vi "Init.vi"(8 "error in (no error)":errorcluster, 11 "PongSwitch in":refnum<class "SnakeSwitch.lvclass">) -> (0 "error out":errorcluster, 3 "PongSwitch out":refnum<class "SnakeSwitch.lvclass">)   [LabVIEW 2019, in "RT_Game.lvlib" / "SnakeSwitch.lvclass"]
uses:
  SnakeSwitch.lvclass
  C:/Users/FreshBob/Dropbox/VIs/myRIO_GameConsole/RT/RT_Game/GameObject/GameObject.lvclass
  Game/Coordinate.ctl
  GameObject/GameObject.lvclass/GameObject.ctl
  GameObject/Write size.vi
  GameObject/Read IsActive.vi
  GameObject/GameObject.lvclass
  Game/Game.lvclass
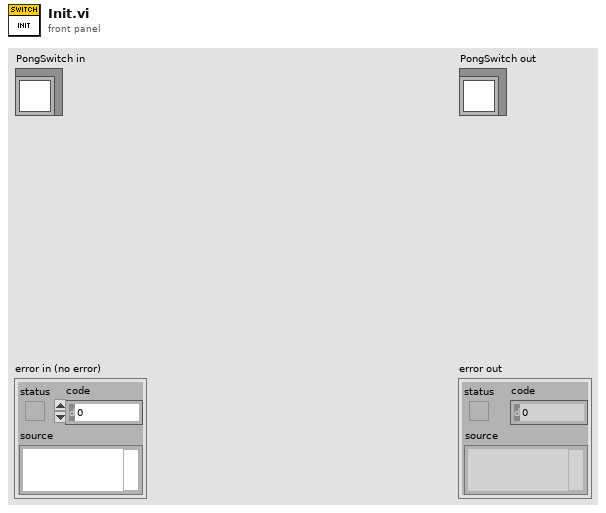
[diagram p1: front panel]
types:
  T1 = typedef "RT_Game.lvlib/Game.lvclass/Coordinate.ctl" = cluster{"x":dbl, "y":dbl}
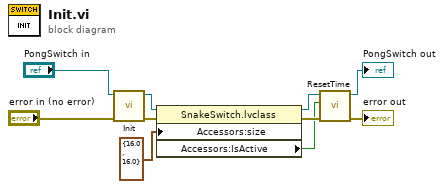
[diagram p0: block diagram]
diagram:
  n1 = call-parent "Init.vi"("error in (no error)"="error in (no error)", "GameObject in"="PongSwitch in") -> ("error out"=w10:errorcluster, "GameObject out"=w6:refnum<class "SnakeSwitch.lvclass">)  [unwired: 8 in]
  n2 = property class="SnakeSwitch.lvclass"(reference=w6, error in=w10, "Accessors:size"=T1 {"x"=16.0, "y"=16.0} ("size")) -> (reference out=w3:refnum<class "SnakeSwitch.lvclass">, error out=w7:errorcluster, "Accessors:IsActive"=w1:bool)
  n3 = call "ResetTime.vi"("error in (no error)"=w7, "enabled"=w1, "SnakeSwitch in"=w3) -> ("error out"=→"error out":errorcluster, "SnakeSwitch out"=→"PongSwitch out":refnum<class "SnakeSwitch.lvclass">)  [unwired: 7 in]
